vi "update_version.vi"(8 "error in (no error)":errorcluster, 9 "commit_hash":string, 10 "version":string, 11 "version_vi":path) -> (0 "error out":errorcluster)   [LabVIEW 2015, in "lv-builder-default.lvlib"]
uses:
  lv-builder-default.lvlib
  <vilib>/Utility/Data Type/NI_Data Type.lvlib
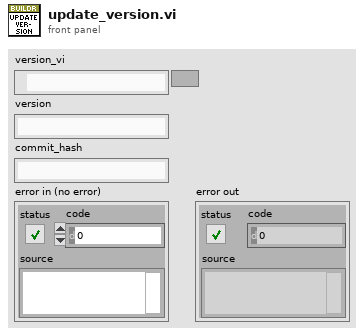
[diagram p1: front panel]
types:
  T1 = typedef "NI_Data Type.lvlib/Data Type.ctl" = enum8{"Invalid Type", "Void", "I8", "I16", "I32", "I64", "U8", "U16", "U32", "U64", "Single Float", "Double Float", "Extended Float", "Single Complex", "Double Complex", "Extended Complex", "Enum U8", "Enum U16", "Enum U32", "Enum U64", "Single Float With Unit", "Double Float With Unit", "Extended Float With Unit", "Single Complex with Unit", "Double Complex with Unit", "Extended Complex with Unit", "Boolean", "String", "Path", "Picture", "Tag", "Array", "Cluster", "Variant", "LV Variant", "Waveform", "Timestamp", "Digital Waveform", "Digital Data", "ExpressData", "Refnum", "External Data", "VI", "Poly VI", "LabVIEW Class Instance", "Fixed Point"}
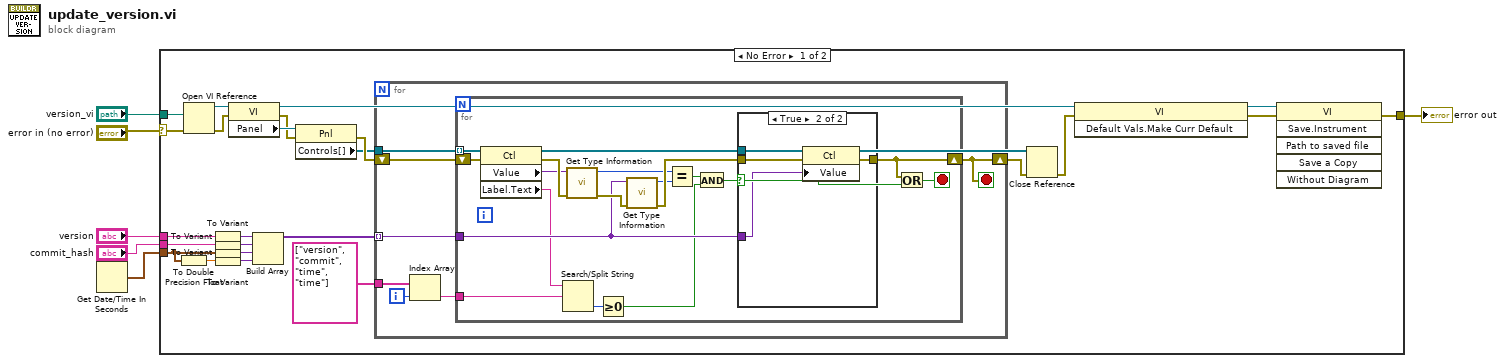
[diagram p0: block diagram]
diagram:
  n1 = Get Date/Time In Seconds() -> (seconds since 1Jan1904=w1:timestamp)
  n2 = case shown="No Error" "error in (no error)" {
    selector: "error in (no error)" -> [w26 w61]
    tunnel: [w22 w61] -> w6
    tunnel: "version_vi" -> [w27 _]
    tunnel: "version" -> [w14 _]
    tunnel: "commit_hash" -> [w9 _]
    tunnel: w1 -> [w8 _]
    frame No Error {
      n3 = To Double Precision Float(number=w8) -> (double precision float=w7:dbl)
      n4 = Open VI Reference(vi path=w27, error in (no error)=w26) -> (vi reference=w21:refnum<vi>, error out=w20:errorcluster)  [unwired: 4 in]
      n5 = To Variant(anything=w14) -> (Variant=w13:variant)
      n6 = To Variant(anything=w9) -> (Variant=w12:variant)
      n7 = To Variant(anything=w8) -> (Variant=w11:variant)
      n8 = To Variant(anything=w7) -> (Variant=w10:variant)
      n9 = property class="VI"(reference=w21, error in=w20) -> (reference out=w25:refnum<vi>, error out=w29:errorcluster, "Panel"=w30:refnum<vi>)
      n10 = Build Array(w13, w12, w11, w10) -> (w19:variant[])
      n11 = property class="Pnl"(reference=w30, error in=w29) -> (error out=w28:errorcluster, "Controls[]"=w17:refnum<vi>[])  [unwired: 1 out]
      n12 = for {
        tunnel: w17 -> [w37]
        tunnel: w19 -> [w35] mode=indexing
        tunnel: string[] ["version", "commit", "time", "time"] -> [w33]
        shift-right: [w34] -> w16
        shift-left: w28 -> [w36]
        i -> [w31]
        stop <- w34 stop-if-true
        n13 = Index Array(array=w33, index=w31) -> (element=w32:string)
        n14 = for {
          tunnel: w37 -> [w53] mode=indexing
          shift-right: [w49] -> w34
          shift-left: w36 -> [w50]
          tunnel: w35 -> [w46]
          tunnel: w32 -> [w48]
          stop <- w47 stop-if-true
          n15 = property class="Ctl"(reference=w53, error in=w50) -> (reference out=w51:refnum<vi>, error out=w54:errorcluster, "Value"=w45:variant, "Label.Text"=w38:string)
          n16 = Search/Split String(string=w38, search string/char (-)=w48) -> (offset of match=w52:i32)  [unwired: 1 in, 2 out]
          n17 = call <vilib>:"Get Type Information.vi"("error in (no error)"=w54, "Variant"=w45) -> ("error out"=w55:errorcluster, "Type"=w43:T1)  [unwired: 5 in, 3 out]
          n18 = Greater Or Equal To 0?(x=w52) -> (x >= 0?=w40:bool)
          n19 = call <vilib>:"Get Type Information.vi"("error in (no error)"=w55, "Variant"=w46) -> ("error out"=w44:errorcluster, "Type"=w42:T1)  [unwired: 5 in, 3 out]
          n20 = Equal?(x=w43, y=w42) -> (x = y?=w41:bool)
          n21 = And(x=w41, y=w40) -> (x .and. y?=w39:bool)
          n22 = case shown="True" w39 {
            tunnel: w51 -> [_ w60]
            tunnel: w44 -> [w56 w59]
            tunnel: [w56 w58] -> w49
            tunnel: w46 -> [_ w57]
            frame False {
            }
            frame True {
              n23 = property class="Ctl"(reference=w60, error in=w59, "Value"=w57) -> (error out=w58:errorcluster)  [unwired: 1 out]
            }
          }
          n24 = Or(x=w49, y=w39) -> (x .or. y?=w47:bool)
        }
      }
      n25 = Close Reference(reference=w17, error in (no error)=w16) -> (error out=w15:errorcluster)
      n26 = invoke class="VI" method="Default Vals.Make Curr Default"(reference=w25, error in=w15) -> (reference out=w23:refnum<vi>, error out=w24:errorcluster)  [unwired: 1 in, 1 out]
      n27 = invoke class="VI" method="Save.Instrument"(reference=w23, error in=w24) -> (error out=w22:errorcluster)  [unwired: 4 in, 5 out]
    }
    frame Error {
    }
  }
  "error out" <- w6
